vi "X-Parker_Plot.vi"(1 "Route Checking?":bool, 3 "Traverse Name":string, 5 "Coordinate rotation (deg)":dbl format="%.2f", 9 "Points to plot":dbl[][](array[numeric]) format="%.2f", 11 "Work in Tunnel Coordinates?":T1, 13 "Speed Factor":dbl=1.0 min=0.1 max=5.0 format="%.2f") -> (4 "Position Output XYZ":dbl[](array[numeric]) format="%.2f", 15 "Error String":string)   [LabVIEW 2010]
uses:
  Gen Trav/Trav_mode.ctl
  ADAM Serial/Instrument drivers/PARKER X/~subVIs/X-_Channel_Config_Global.vi
  Globals/Trav_pos_global.vi
  ADAM Client/Sub VIs/ADAM Controls/Update_scan_value.ctl
  Gen Trav/Route mapping/Route_mapping_global.vi
  Globals/Preference_global.vi
  Controls/Tunnel_Coordinates.ctl
panel:
  out "Server copy Location":path
  in  "Backlash Compensation?":bool
  out "Log File":path
  out "Achieved Pos In Eng units of all channels":dbl[](array[numeric]) format="%.2f"
  out "Pulses Positon all channels":dbl[](array[numeric])
  out "Counters Reset?":bool
  in  "Mode":T2
  # "X                Y                   Z"
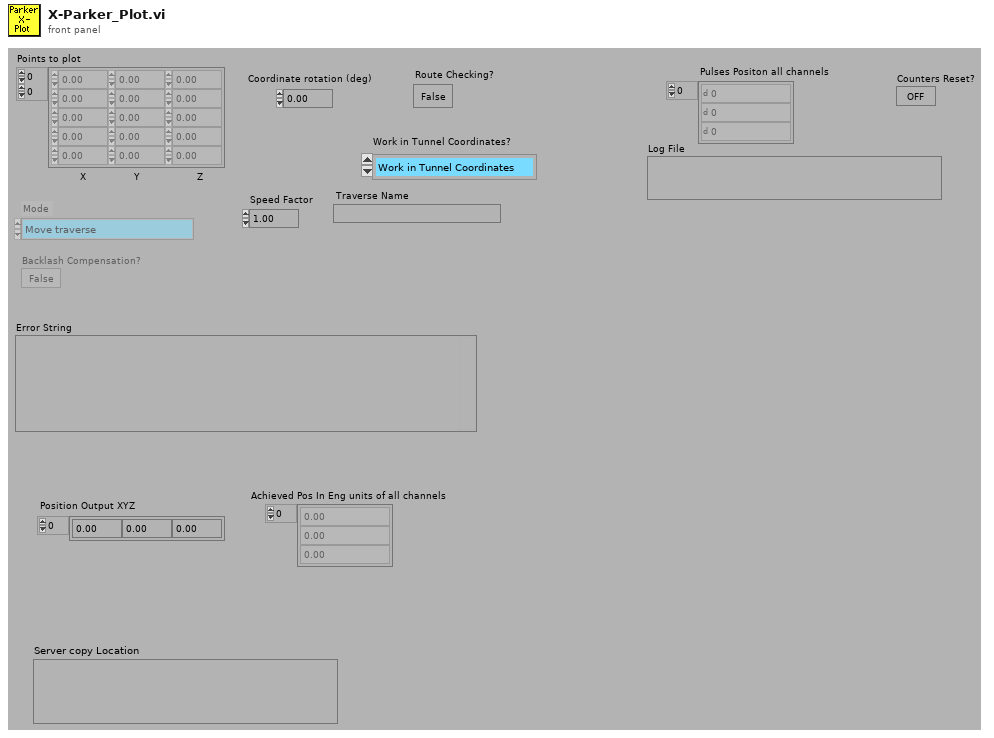
[diagram p1: front panel]
types:
  T1 = typedef "Tunnel_Coordinates.ctl" = enum16{"Work in Tunnel Coordinates", "Work in Model Coordinates"}
  T2 = typedef "Trav_mode.ctl" = enum16{"Move traverse", "Read traverse position", "Teach Position"}
  T3 = enum16{"A-    Acceleration (rps)", "B-    Buffer Status", "C-    Continue", "CG-  Correction Gain", "CR-  Cariage Return", "D-    Distance (pulses)", "DB-  Dead Band (encoder steps)", "DW- Deadband Window (encoder steps)", "E-    Enable Communications", "ER-  Encoder Resolution (steps/rev)", "F-    Disable Communications", "FS-  Encoder Functions Report", "FSA- Incremental/Absolute (0/1)", "FSB- Motor/Encoder Step Mode (0/1)", "FSC- Enable/Disable Position Maint. (1/0)", "FSD- Stop/Continue on Stall (1/0)", "FSE- Activate o/p1 on Stall (1/0)", "FSF- Stop Motion on Trig3 (1/0)", "FSG- Activate o/p2 in Deadband (1/0)", "FSH- Enable Stall Detect (1/0)", "G- Go", "GH- Go Home and Zero (+/-V)", "^H- Delete ", "H- Direction Reverse/CCW/CW (0,1,2)", "IS- Input Status", "K- Kill", "L- Loop (n)", "LD- Limit DISABLE (0-none,1-CW,2-CCW,3-Both)", "LF- Line Feed", "MC- Mode Continuous", "MN- Mode Normal", "MPA- Motor Postion Absolute", "MPI- Motor Position Incremental", "MR- Motor Resolution (Drive Steps/rev)", "N- End of Loop", "O- Output (00,01,10,11)", "OS- Report Homing Setup", "OSA- NO/NC Limits (1/0)", "OSB- Back Up to Home/Edge? (0/1)", "OSC- NO/NC Home Switch (1/0)", "OSD- Enable Encoder Z for Home (0/1)", "OSH- Reference Edge for Home CW/CCW (0/1)", "PR- Report ABSOLUTE Position", "PS- Pause until Continue", "PX- Report Absolute ENCODER Position", "PZ- Zero Absolute Counter", "\"- Quote (17 ASCII +Space)", "Q- Enter/Exit Velocity Profiling (1/0)", "R- Request Indexer Status", "RA- Report Limit Switch Status", "RB- Report Loop, Pause, Shutdown, Trigger Status", "RC- Report Closed Loop Status", "RM- Velocity Streaming Rate Multiplier (000-FFF)", "RV- Report Revision Level", "S- Controlled Stop", "SN- Debounce (1-1000ms)", "SS- Report Software Switch Status", "SSA- Disable RS232 Echo (1/0)", "SSG- Clear/Save Command Buffer on Limit (0/1)", "SSH- Clear/Save Command Buffer on Stop (0/1)", "ST- Shutdown (1/0)", "SV- Servoing Setting (0,1,2,3)", "T- Time Delay (0.01-99999.99)", "TR- Wait for Trigger High/Low/Ignore (1/0/X)", "TS- Report Trigger Status", "U- Pause after Move Until Continue", "V- Velocity (0.01-50.00 revs/sec)", "W1- Report Relative Position <Signed Binary>", "W3- Report Relative Position <Hexadecimal>", "Y- Abort Loop at N", "Z-    Reset to Defaults", "#-    Disable/Set Soft Addresses (0/1-255)"}
  T4 = enum16{"To Traverse Coordinates", "To User Coordinates"}
  T5 = typedef "Update_scan_value.ctl" = cluster{"Channel Name":string, "New Value":dbl}
  T6 = typedef "X-Config_Cluster.ctl" = cluster{"Channel Properties":T7, "Static Drive Configuration":T8}
  T7 = typedef "Ch_Properties.ctl" = cluster{"Channel Name":string, "Vel. Default":dbl, "Acc. Default":dbl, "Vel. Max":dbl, "Vel. Min":dbl, "Acc. Max":dbl, "Acc. Min":dbl, "Pulses/unit":dbl, "Address":u8, "Pulse Offset":i32, "Pos Tolerance":dbl, "Pulses/rev":dbl, "Backlash/Eng units":dbl, "Current Pos":dbl, "Ch Status":enum16{"Active", "Offline", "Simulate"}, "Port Name":string, "Axis Transform mode":string, "Metadata Ch Name":string}
  T8 = typedef "X-_Static_Config.ctl" = cluster{"Correction Gain % (CG)":u16, "Dead Band (DB)":i32, "Dead Band Window (DW)":i32, "Encoder Resolution (ER)":i32, "Step Mode  (FSB)":u16, "Position Maintenance (FSC)":u16, "Stop on Stall (FSD)":u16, "Activate OP1 on stall (FSE)":u16, "Stop on Trigger 3 (FSF)":u16, "OP2 in Deadband (FSG)":u16, "Stall Detect (FSH)":u16, "Limit Disable (LD)":u16, "Motor Resolution (MR)":enum16{"200", "400", "1000", "2000", "4000", "5000", "10000", "12800", "18000", "20000", "21600", "25000", "25400", "25600", "36000", "50000", "278528", "425984", "507904", "614400", "655360", "819200", "1024000"}, "Limit Switch Sense (OSA)":u16, "Home Position (OSB)":u16, "Home Switch Sense (OSC)":u16, "Encoder Z for Home (OSD)":u16, "Reference edge of Home (OSH)":u16, "RS232 Echo Control (SSA)":u16, "Buffer at Limit (SSG)":u16, "Buffer at Stop (SSH)":u16, "Indexer Mode  (FSA)":u16}
  T9 = typedef "Box_size.ctl" = cluster{"Max":dbl, "Min":dbl}[]
  T10 = typedef "Exclude_cluster.ctl" = cluster{"Sizes":T9, "Name":string, "Exclude Type":T11}
  T11 = typedef "Exclusion_type.ctl" = enum16{"Exclude completely", "Allow only vertical moves"}
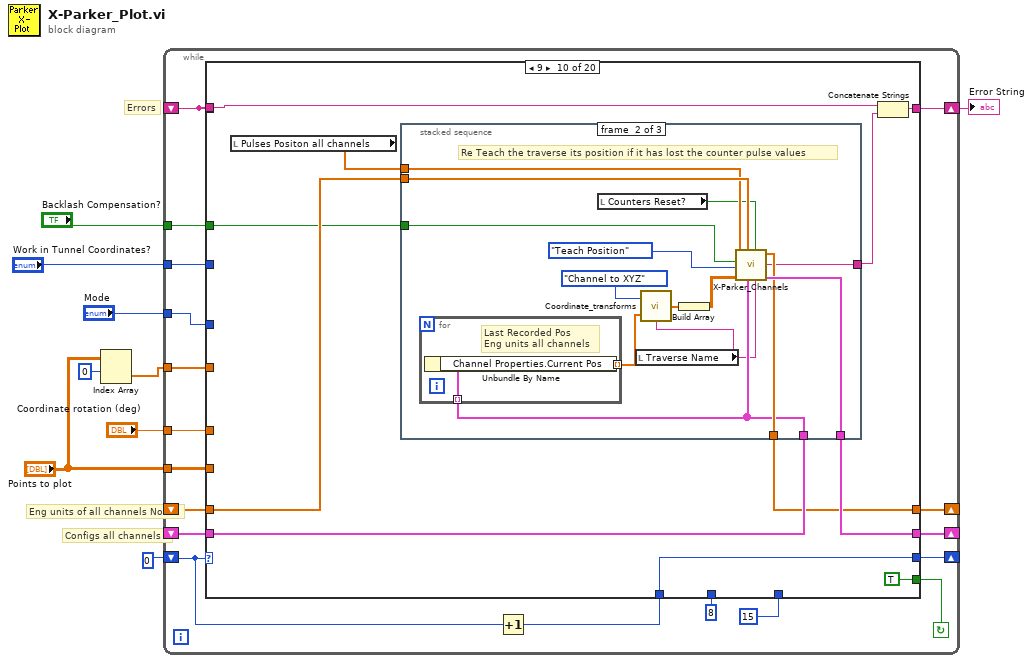
[diagram p0: block diagram]
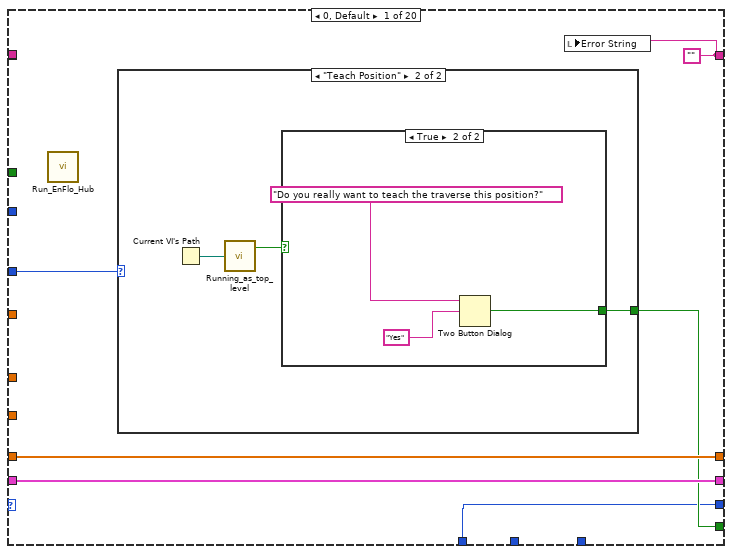
[diagram p2: hidden frame]
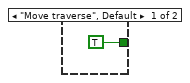
[diagram p3: hidden frame]
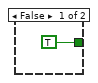
[diagram p4: hidden frame]
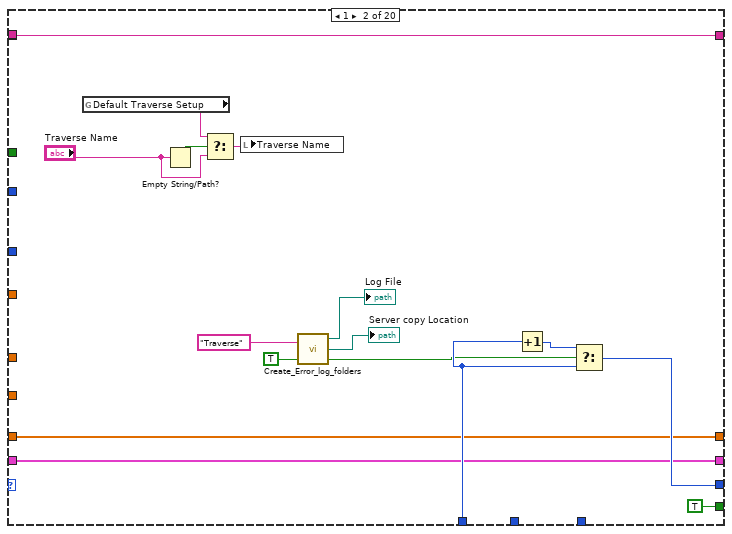
[diagram p5: hidden frame]
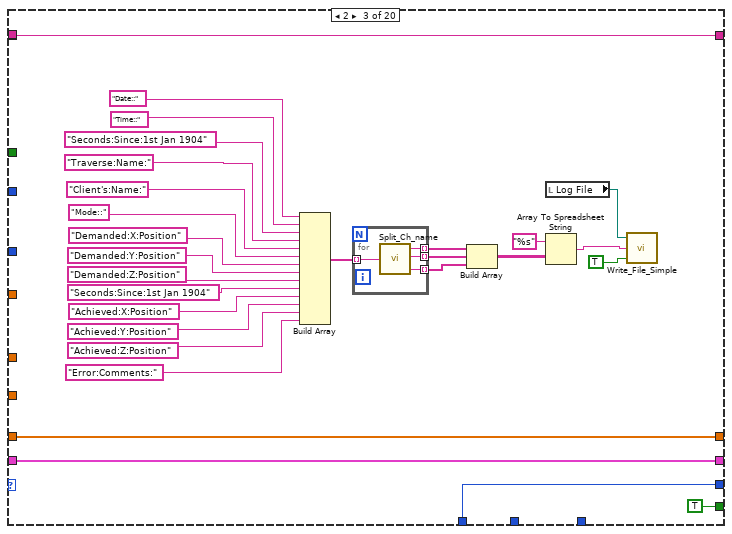
[diagram p6: hidden frame]
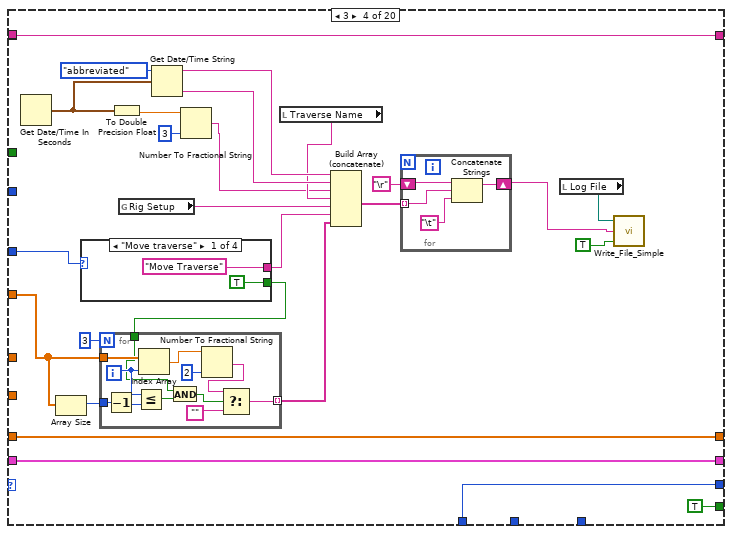
[diagram p7: hidden frame]
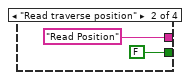
[diagram p8: hidden frame]
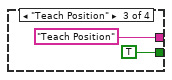
[diagram p9: hidden frame]
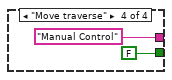
[diagram p10: hidden frame]
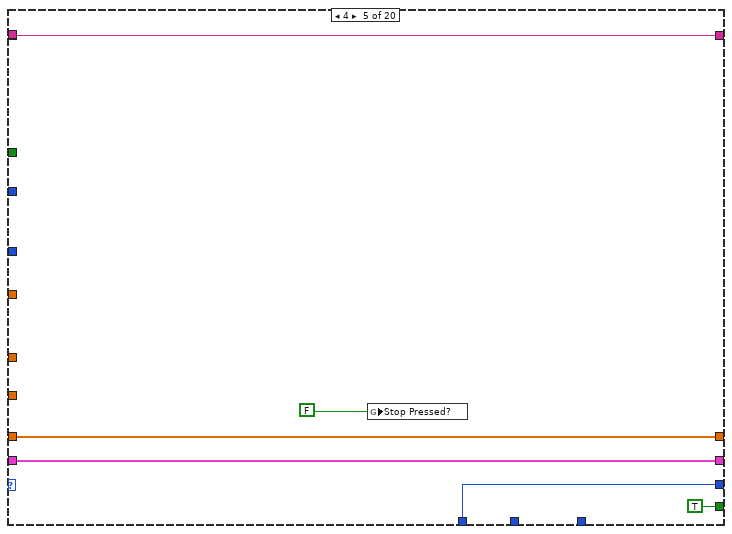
[diagram p11: hidden frame]
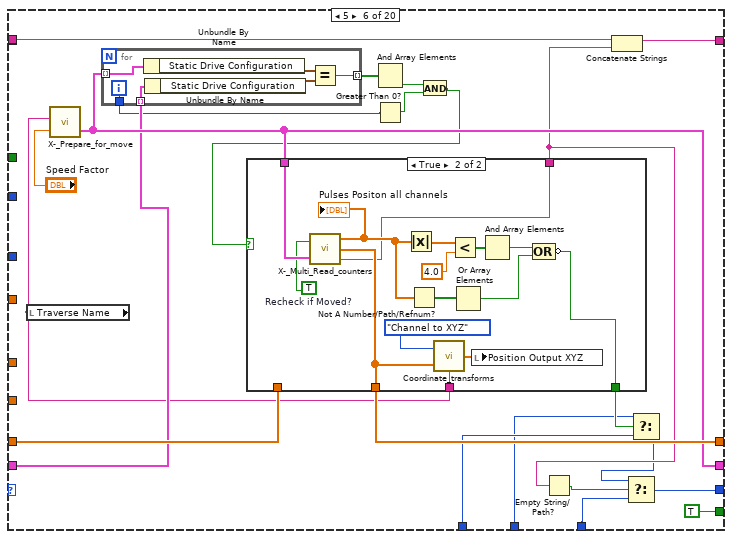
[diagram p12: hidden frame]
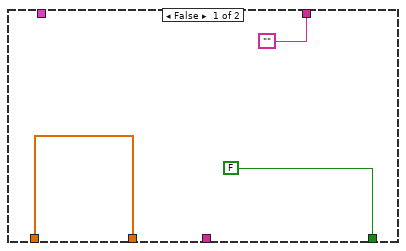
[diagram p13: hidden frame]
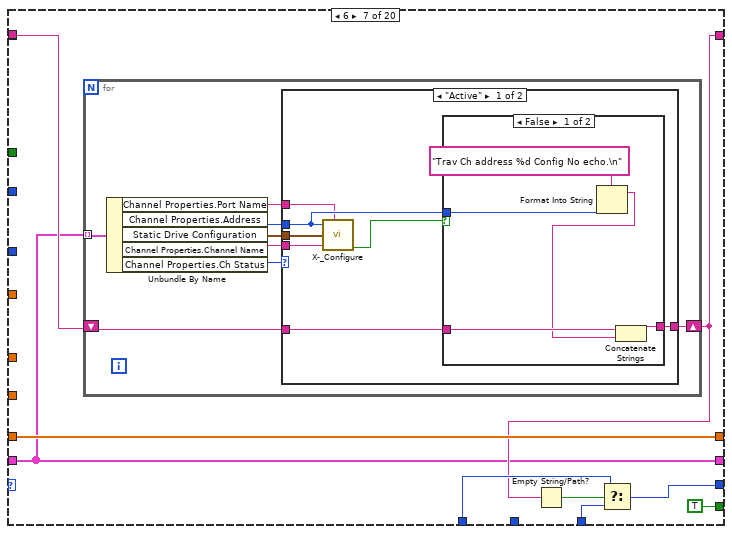
[diagram p14: hidden frame]
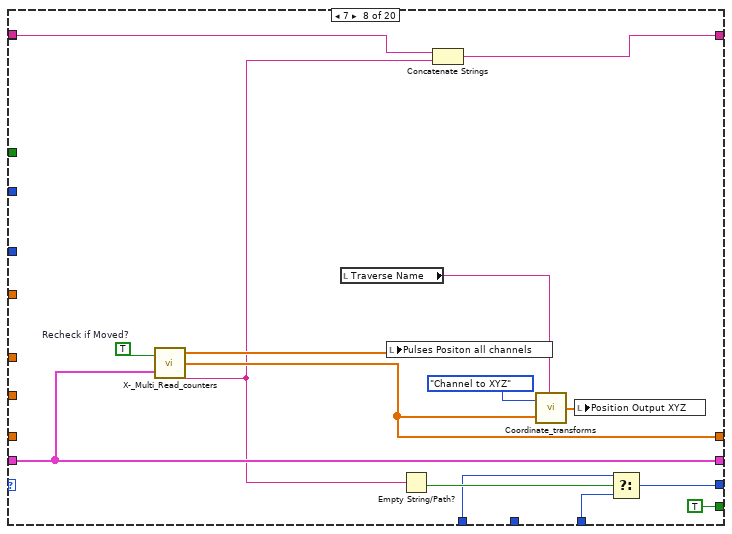
[diagram p17: hidden frame]
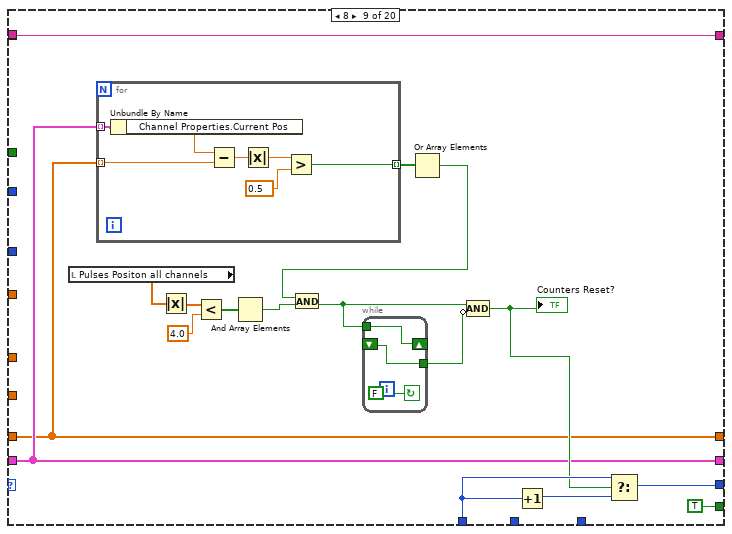
[diagram p18: hidden frame]
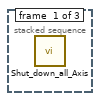
[diagram p19: hidden frame]
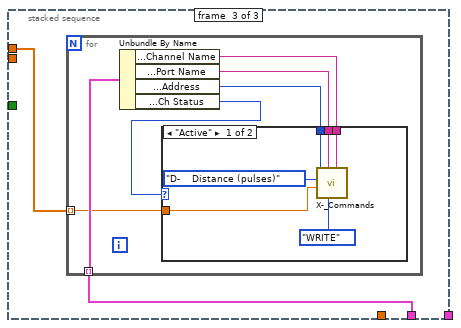
[diagram p20: hidden frame]
diagram:
  # "Errors"
  # "Eng units of all channels Now"
  # "Configs all channels"
  n1 = Index Array(array="Points to plot", index (row)=0) -> (element=w2:dbl[])  [unwired: 1 in]
  n2 = while {
    tunnel: "Backlash Compensation?" -> [w13]
    tunnel: w2 -> [w17]
    shift-left: _ -> [w14]
    shift-right: [w18] -> w7
    shift-left: _ -> [w19]
    shift-right: [w20] -> _
    shift-left: _ -> [w21]
    shift-right: [w22] -> _
    shift-left: 0 -> [w25]
    shift-right: [w23] -> _
    tunnel: "Mode" -> [w27]
    tunnel: "Coordinate rotation (deg)" -> [w12]
    tunnel: "Work in Tunnel Coordinates?" -> [w11]
    tunnel: "Points to plot" -> [w10]
    stop <- w26 continue-if-true
    n3 = Increment(x=w25) -> (x+1=w24:i32)
    n4 = case shown="9" w25 {
      tunnel: w27 -> [w33 _ _ w108 _ _ _ _ _ _ w311 _ w389 w405 _ _ _ w477 _ w533]
      tunnel: [w30 TRUE ("T button?") TRUE ("T button?") TRUE ("T button?") TRUE TRUE ("T button?") TRUE ("T button?") TRUE ("T button?") TRUE TRUE TRUE ("T button?") TRUE ("T button?") TRUE TRUE TRUE ("T button?") TRUE ("T button?") TRUE ("T button?") w479 TRUE FALSE] -> w26
      tunnel: w24 -> [w29 w56 w65 w113 w140 w164 w197 w225 w250 w266 w310 w343 w380 w407 w429 w443 w472 w476 w511 w540]
      tunnel: [w29 w54 w65 w113 w140 w147 w196 w223 w248 w266 w309 w344 w380 w406 w429 w441 w472 w475 w511 w540] -> w23
      tunnel: [w31 w51 w67 w115 w142 w162 w192 w237 w244 w275 w307 w346 w374 w404 w431 w455 w474 w482 w509 w538] -> w22
      tunnel: w21 -> [w31 w51 w67 w115 w142 w161 w192 w237 w244 w274 w307 w346 w387 w404 w431 w455 w474 w482 w509 w538]
      tunnel: [w32 w52 w66 w114 w143 w167 w200 w232 w243 w271 w306 w333 w381 w410 w430 w454 w473 w483 w512 w541] -> w20
      tunnel: w19 -> [w32 w52 w66 w114 w143 w166 w200 _ w243 w272 w306 w333 w376 w410 w430 w454 w473 w483 w512 w541]
      tunnel: [w28 w50 w63 w105 w144 w152 w193 w228 w247 w268 w312 w337 w383 w408 w427 w445 w470 w478 w505 w534] -> w18
      tunnel: w14 -> [_ w50 w63 w105 w144 w153 w194 w229 w247 w270 w312 _ w384 w408 w427 w445 w470 w481 w507 w536]
      tunnel: w17 -> [_ _ _ w102 _ _ _ _ _ _ _ _ _ _ _ _ _ _ w503 _]
      tunnel: 15 ("f") -> [_ _ _ _ _ w148 w195 w224 _ _ _ w339 _ _ _ _ _ _ _ _]
      tunnel: 8 ("t") -> [_ _ _ _ _ w163 _ _ _ _ _ _ _ _ _ _ _ _ _ _]
      tunnel: w14 -> [_ _ _ _ _ _ _ _ _ _ _ w340 _ _ _ _ _ _ _ _]
      tunnel: w13 -> [_ _ _ _ _ _ _ _ _ w265 _ _ w375 w399 _ _ _ _ _ _]
      tunnel: w12 -> [_ _ _ _ _ _ _ _ _ _ _ w332 w372 _ _ _ _ _ w504 w531]
      tunnel: w11 -> [_ _ _ _ _ _ _ _ _ _ _ _ w373 _ _ _ _ _ w501 w529]
      tunnel: w10 -> [_ _ _ _ _ _ _ _ _ _ _ w325 w371 _ _ _ _ _ _ _]
      frame 0, Default {
        w28 = ""
        n5 = call "Run_EnFlo_Hub.vi"() -> ()  [unwired: 8 in]
        n6 = case shown="\"Teach Position\"" w33 {
          tunnel: [TRUE ("T button?") w35] -> w30
          frame "Move traverse", Default {
          }
          frame "Teach Position" {
            n7 = Current VI's Path() -> (path=w37:path)
            n8 = call "Running_as_top_level.vi"("Vi path name"=w37) -> ("Top Level"=w36:bool)  [unwired: 1 out]
            n9 = case shown="True" w36 {
              tunnel: [TRUE ("T button?") w39] -> w35
              frame False {
              }
              frame True {
                n10 = Two Button Dialog(message="Do you really want to teach the traverse this position?", 2:"Yes" ("T button name (\"OK\")")) -> (T button?=w39:bool)  [unwired: 1 in]
              }
            }
          }
        }
        n11 = local write "Error String"(w28) -> ()
      }
      frame 1 {
        n12 = global read "Trav_pos_global.vi" "Default Traverse Setup"() -> (w47:string)
        n13 = Empty String/Path?(string/path="Traverse Name") -> (empty?=w45:bool)
        n14 = Select(t=w47, s=w45, f="Traverse Name") -> (s? t:f=w44:string)
        n15 = local write "Traverse Name"(w44) -> ()
        n16 = call "Create_Error_log_folders.vi"("Per Day Log File?"=TRUE, "Log Filename"="Traverse" ("Input Element")) -> ("exists?"=w48:bool, "Server copy Location"=→"Server copy Location":path, "Local Log File"=→"Log File":path)  [unwired: 1 in]
        n17 = Increment(x=w56) -> (x+1=w55:i32)
        n18 = Select(t=w55, s=w48, f=w56) -> (s? t:f=w54:i32)
      }
      frame 2 {
        n19 = Build Array("Date::", "Time::", "Seconds:Since:1st Jan 1904", "Traverse:Name:", "Client's:Name:", "Mode::", "Demanded:X:Position", "Demanded:Y:Position", "Demanded:Z:Position", "Seconds:Since:1st Jan 1904", "Achieved:X:Position", "Achieved:Y:Position", "Achieved:Z:Position", "Error:Comments:") -> (w70:string[])
        n20 = for {
          tunnel: w70 -> [w89] mode=indexing
          tunnel: [w88] -> w71 mode=indexing
          tunnel: [w87] -> w72 mode=indexing
          tunnel: [w86] -> w73 mode=indexing
          n21 = call "Split_Ch_name.vi"("Ch name"=w89) -> ("Top level"=w88:string, "Middle"=w87:string, "Low level"=w86:string)
        }
        n22 = Build Array(w71, w72, w73) -> (w68:string[][])
        n23 = local read "Log File"() -> (w59:path)
        n24 = Array To Spreadsheet String(array=w68, 3:"%s" ("format string")) -> (spreadsheet string=w60:string)  [unwired: 1 in]
        n25 = call "Write_File_Simple.vi"("append to file? (new file:F)"=TRUE, "character string"=w60, "file path"=w59) -> ()  [unwired: 2 out]
      }
      frame 3 {
        n26 = Get Date/Time In Seconds() -> (seconds since 1Jan1904=w94:timestamp)
        n27 = Array Size(array=w102) -> (size(s)=w103:i32)
        n28 = case shown="\"Move traverse\"" w108 {
          tunnel: ["Move Traverse" "Read Position" "Teach Position" "Manual Control"] -> w109
          tunnel: [TRUE FALSE TRUE FALSE] -> w99
          frame "Move traverse" {
          }
          frame "Read traverse position" {
          }
          frame "Teach Position" {
          }
          frame "Move traverse" {
          }
        }
        n29 = for {
          N: 3 -> [_]
          tunnel: w102 -> [w127]
          tunnel: w103 -> [w124]
          tunnel: [w120] -> w100 mode=indexing
          tunnel: w99 -> [w116]
          i -> [w122]
          n30 = Decrement(x=w124) -> (x-1=w123:i32)
          n31 = Less Or Equal?(x=w122, y=w123) -> (x <= y?=w118:bool)
          n32 = Index Array(array=w127, index=w122) -> (element=w126:dbl)
          n33 = And(x=w116, y=w118) -> (x .and. y?=w117:bool)
          n34 = Number To Fractional String(number=w126, precision (6)=i16 2) -> (F-format string=w121:string)  [unwired: 2 in]
          n35 = Select(t=w121, s=w117, f="") -> (s? t:f=w120:string)
        }
        n36 = To Double Precision Float(number=w94) -> (double precision float=w93:dbl)
        n37 = global read "Preference_global.vi" "Rig Setup"() -> (w90:string)
        n38 = Get Date/Time String(date format (0)=enum16{"short", "long", "abbreviated"}."abbreviated", seconds (now)=w94) -> (date string=w111:string, time string=w110:string)  [unwired: 1 in]
        n39 = Number To Fractional String(number=w93, precision (6)=i16 3) -> (F-format string=w91:string)  [unwired: 2 in]
        n40 = local read "Traverse Name"() -> (w95:string)
        n41 = Build Array (concatenate)(w111, w110, w91, w95, w90, w109, w100) -> (w106:string[])
        n42 = for {
          shift-right: [w130] -> w96
          shift-left: "\r" -> [w131]
          tunnel: w106 -> [w129] mode=indexing
          n43 = Concatenate Strings(w131, w129, "\t") -> (w130:string)
        }
        n44 = local read "Log File"() -> (w97:path)
        n45 = call "Write_File_Simple.vi"("append to file? (new file:F)"=TRUE, "character string"=w96, "file path"=w97) -> ()  [unwired: 2 out]
      }
      frame 4 {
        n46 = global write "X-_Channel_Config_Global.vi" "Stop Pressed?"(FALSE) -> ()
      }
      frame 5 {
        n47 = local read "Traverse Name"() -> (w155:string)
        n48 = call "X-_Prepare_for_move.vi"("Speed Factor"="Speed Factor", "Traverse Name"=w155) -> ("Matched Configurations"=w162:T6[])  [unwired: 1 in]
        n49 = for {
          tunnel: w162 -> [w173] mode=indexing
          tunnel: w161 -> [w172] mode=indexing
          tunnel: [w169] -> w160 mode=indexing
          tunnel: [w168] -> w159
          i -> [w168]
          n50 = Unbundle By Name(w173) -> ("Static Drive Configuration"=w171:T8)
          n51 = Unbundle By Name(w172) -> ("Static Drive Configuration"=w170:T8)
          n52 = Equal?(x=w171, y=w170) -> (x = y?=w169:bool)
        }
        n53 = And Array Elements(Boolean array=w160) -> (logical AND=w157:bool)
        n54 = Greater Than 0?(x=w159) -> (x > 0?=w158:bool)
        n55 = And(x=w157, y=w158) -> (x .and. y?=w156:bool)
        n56 = case shown="True" w156 {
          tunnel: w162 -> [_ w191]
          tunnel: [w176 w181] -> w167
          tunnel: w166 -> [w176 _]
          tunnel: [FALSE w183] -> w165
          tunnel: w155 -> [_ w179]
          tunnel: ["" w177] -> w151
          frame False {
          }
          frame True {
            w178 = TRUE  # Recheck if Moved?
            n57 = call "X-_Multi_Read_counters.vi"("Recheck if Moved?"=w178, "Matched Configurations"=w191) -> ("Pulses"=w186:dbl[], "Eng units"=w181:dbl[], "Error String"=w177:string)
            "Pulses Positon all channels" <- w186
            n58 = Absolute Value(x=w186) -> (abs(x)=w190:dbl[])
            n59 = Not A Number/Path/Refnum?(number/path/refnum=w186) -> (NaN/Path/Refnum?=w185:bool[])
            n60 = call "Coordinate_transforms.vi"("Traverse Name"=w179, "Input"=w181, "Mode"=enum16{"XYZ to Channel", "Channel to XYZ"}."Channel to XYZ") -> ("Output"=w180:dbl[])
            n61 = Less?(x=w190, y=4.0 ("Achieved Position")) -> (x < y?=w188:bool[])
            n62 = Or Array Elements(Boolean array=w185) -> (logical OR=w184:bool)
            n63 = local write "Position Output XYZ"(w180) -> ()
            n64 = And Array Elements(Boolean array=w188) -> (logical AND=w187:bool)
            n65 = Compound Arithmetic op=OR(w187, w184) -> (invert w183:bool)
          }
        }
        n66 = Empty String/Path?(string/path=w151) -> (empty?=w150:bool)
        n67 = Concatenate Strings(w153, w151) -> (w152:string)
        n68 = Select(t=w163, s=w165, f=w164) -> (s? t:f=w149:i32)
        n69 = Select(t=w149, s=w150, f=w148) -> (s? t:f=w147:i32)
      }
      frame 6 {
        n70 = for {
          tunnel: w192 -> [w208] mode=indexing
          shift-right: [w201] -> w193
          shift-left: w194 -> [w202]
          n71 = Unbundle By Name(w208) -> ("Channel Properties.Port Name"=w203:string, "Channel Properties.Address"=w207:u8, "Static Drive Configuration"=w206:T8, "Channel Properties.Channel Name"=w205:string, "Channel Properties.Ch Status"=w204:enum16{"Active", "Offline", "Simulate"})
          n72 = case shown="\"Active\"" w204 {
            tunnel: w207 -> [w213 _]
            tunnel: w206 -> [w215 _]
            tunnel: w205 -> [w214 _]
            tunnel: w203 -> [w212 _]
            tunnel: w202 -> [w210 w222]
            tunnel: [w209 w222] -> w201
            frame "Active" {
              n73 = call "X-_Configure.vi"("Address"=w213, "Port Name"=w212, "Static Drive Configuration"=w215, "Channel Name"=w214) -> ("Good Echo"=w211:bool)  [unwired: 4 in]
              n74 = case shown="False" w211 {
                tunnel: w213 -> [w220 _]
                tunnel: w210 -> [w218 w221]
                tunnel: [w217 w221] -> w209
                frame False {
                  n75 = Format Into String(format string="Trav Ch address %d Config No echo.\n" ("Format String"), w220) -> (resulting string=w216:string)  [unwired: 2 in, 1 out]
                  n76 = Concatenate Strings(w218, w216) -> (w217:string)
                }
                frame True {
                }
              }
            }
            frame "Offline", Default {
            }
          }
        }
        n77 = Empty String/Path?(string/path=w193) -> (empty?=w198:bool)
        n78 = Select(t=w197, s=w198, f=w195) -> (s? t:f=w196:i32)
      }
      frame 7 {
        w230 = TRUE  # Recheck if Moved?
        n79 = call "X-_Multi_Read_counters.vi"("Recheck if Moved?"=w230, "Matched Configurations"=w237) -> ("Pulses"=w235:dbl[], "Eng units"=w232:dbl[], "Error String"=w226:string)
        n80 = local read "Traverse Name"() -> (w231:string)
        n81 = local write "Pulses Positon all channels"(w235) -> ()
        n82 = Empty String/Path?(string/path=w226) -> (empty?=w227:bool)
        n83 = Concatenate Strings(w229, w226) -> (w228:string)
        n84 = call "Coordinate_transforms.vi"("Traverse Name"=w231, "Input"=w232, "Mode"=enum16{"XYZ to Channel", "Channel to XYZ"}."Channel to XYZ") -> ("Output"=w233:dbl[])
        n85 = local write "Position Output XYZ"(w233) -> ()
        n86 = Select(t=w225, s=w227, f=w224) -> (s? t:f=w223:i32)
      }
      frame 8 {
        n87 = local read "Pulses Positon all channels"() -> (w238:dbl[])
        n88 = for {
          tunnel: w244 -> [w264] mode=indexing
          tunnel: w243 -> [w262] mode=indexing
          tunnel: [w258] -> w241 mode=indexing
          n89 = Unbundle By Name(w264) -> ("Channel Properties.Current Pos"=w263:dbl)
          n90 = Subtract(x=w263, y=w262) -> (x-y=w261:dbl)
          n91 = Absolute Value(x=w261) -> (abs(x)=w260:dbl)
          n92 = Greater?(x=w260, y=0.5) -> (0:w258:bool)
        }
        n93 = Absolute Value(x=w238) -> (abs(x)=w254:dbl[])
        n94 = Less?(x=w254, y=4.0 ("Achieved Position")) -> (x < y?=w252:bool[])
        n95 = And Array Elements(Boolean array=w252) -> (logical AND=w242:bool)
        n96 = Or Array Elements(Boolean array=w241) -> (logical OR=w240:bool)
        n97 = And(x=w240, y=w242) -> (x .and. y?=w239:bool)
        n98 = while {
          tunnel: [w256] -> w246
          tunnel: w239 -> [w257]
          shift-left: _ -> [w256]
          shift-right: [w257] -> _
          stop <- FALSE continue-if-true
        }
        n99 = Compound Arithmetic op=AND(w239, invert w246) -> (w245:bool)
        "Counters Reset?" <- w245
        n100 = Increment(x=w250) -> (x+1=w249:i32)
        n101 = Select(t=w250, s=w245, f=w249) -> (s? t:f=w248:i32)
      }
      frame 9 {
        n102 = local read "Pulses Positon all channels"() -> (w273:dbl[])
        n103 = stacked-sequence {
          tunnel: w273 -> [_ w281 w292]
          tunnel: [_ w289 _] -> w275
          tunnel: w272 -> [_ w288 _]
          tunnel: [_ w287 _] -> w271
          tunnel: w274 -> [_ w283 w293]
          tunnel: [_ w286 _] -> w269
          tunnel: w265 -> [_ w277 _]
          frame #0 {
            n104 = call "Shut_down_all_Axis.vi"() -> ()  [unwired: 1 in]
          }
          frame #1 {
            # "Re Teach the traverse its position if it has lost the counter pulse values"
            n105 = for {
              tunnel: [w291] -> w282 mode=indexing
              tunnel: w283 -> [w290] mode=indexing
              # "Last Recorded Pos\nEng units all channels"
              n106 = Unbundle By Name(w290) -> ("Channel Properties.Current Pos"=w291:dbl)
            }
            n107 = local read "Counters Reset?"() -> (w279:bool)
            n108 = local read "Traverse Name"() -> (w278:string)
            n109 = call "Coordinate_transforms.vi"("Traverse Name"=w278, "Input"=w282, "Mode"=enum16{"XYZ to Channel", "Channel to XYZ"}."Channel to XYZ") -> ("Output"=w284:dbl[])
            n110 = Build Array(w284) -> (w276:dbl[][])
            n111 = call "X-Parker_Channels.vi"("Traverse Name"=w278, "Counters Reset?"=w279, "Matched Configurations all Channels In"=w283, "Current Pos In Eng units of all channels"=w288, "Position Steps"=w276, "Mode"=Trav_mode."Teach Position", "Backlash Compensation?"=w277, "Current Pulses positions for all channels"=w281) -> ("Matched Configurations Out"=w289:T6[], "Error String"=w286:string, "Achieved Pos In Eng units of all channels"=w287:dbl[])  [unwired: 1 in]
          }
          frame #2 {
            n112 = for {
              tunnel: w293 -> [w299] mode=indexing
              tunnel: w292 -> [w296] mode=indexing
              n113 = Unbundle By Name(w299) -> ("Channel Properties.Channel Name"=w294:string, "Channel Properties.Port Name"=w295:string, "Channel Properties.Address"=w298:u8, "Channel Properties.Ch Status"=w297:enum16{"Active", "Offline", "Simulate"})
              n114 = case shown="\"Active\"" w297 {
                tunnel: w295 -> [w305 _]
                tunnel: w294 -> [w304 _]
                tunnel: w298 -> [w301 _]
                tunnel: w296 -> [w300 _]
                frame "Active" {
                  n115 = call "X-_Commands.vi"("Channel Name"=w304, "R/W"=enum16{"READ", "WRITE"}."WRITE", "Port Name"=w305, "Numeric Value"=w300, "COMMAND"=T3."D-    Distance (pulses)", "Address"=w301) -> ()  [unwired: 3 in, 2 out]
                }
                frame "Offline", Default {
                }
              }
            }
          }
        }
        n116 = Concatenate Strings(w270, w269) -> (w268:string)
      }
      frame 10 {
        n117 = case shown="\"Move traverse\"" w311 {
          tunnel: w310 -> [w313 w320]
          tunnel: [w315 w319] -> w309
          frame "Move traverse" {
            n118 = Increment(x=w313) -> (x+1=w314:i32)
            n119 = case shown="True" "Route Checking?" {
              tunnel: [w317 w318] -> w315
              tunnel: w314 -> [w317 _]
              tunnel: w313 -> [_ w318]
              frame False {
              }
              frame True {
              }
            }
          }
          frame "Read traverse position", Default {
            n120 = Increment(x=w320) -> (x+1=w319:i32)
          }
        }
      }
      frame 11 {
        w328 = 0.1  # Reduce by
        n121 = global read "Route_mapping_global.vi" "Probe Volume"() -> (w327:T9)
        n122 = local read "Traverse Name"() -> (w334:string)
        n123 = for {
          tunnel: w327 -> [w369] mode=indexing
          tunnel: [w368] -> w326 mode=indexing
          tunnel: w328 -> [w363]
          n124 = Unbundle By Name(w369) -> ("Max"=w367:dbl, "Min"=w365:dbl)
          n125 = Subtract(x=w367, y=w363) -> (x-y=w366:dbl)
          n126 = Add(x=w363, y=w365) -> (x+y=w364:dbl)
          n127 = Bundle By Name(cluster=w369, "Max"=w366, "Min"=w364) -> (w368:cluster{"Max":dbl, "Min":dbl})
        }
        n128 = global read "Route_mapping_global.vi" "Entire Space"() -> (w329:T9)
        n129 = global read "Route_mapping_global.vi" "Exclude Array"() -> (w330:T10[])
        n130 = call "Coordinate_transforms.vi"("Traverse Name"=w334, "Input"=w333, "Mode"=enum16{"XYZ to Channel", "Channel to XYZ"}."Channel to XYZ") -> ("Output"=w335:dbl[])
        n131 = Array Size(array=w325) -> (size(s)=w324:i32[])
        n132 = Index Array(array=w324, index=0) -> (element=w322:i32)
        n133 = call "Coordinate_rotation.vi"("Input Position"=w335, "Coordinate rotation (deg)"=w332, "Mode"=T4."To User Coordinates") -> ("Output Position"=w341:dbl[])
        n134 = Decrement(x=w322) -> (x-1=w321:i32)
        n135 = while {
          tunnel: w341 -> [w361]
          tunnel: w325 -> [w359] mode=indexing
          tunnel: w334 -> [w358]
          tunnel: w332 -> [w356]
          tunnel: [w352] -> w331
          tunnel: w330 -> [w355]
          tunnel: w329 -> [w354]
          tunnel: w326 -> [w353]
          tunnel: w321 -> [w350]
          i -> [w351]
          stop <- w347 continue-if-true
          w357 = FALSE  # Full Check
          n136 = Less?(x=w351, y=w350) -> (x < y?=w348:bool)
          n137 = call "Coordinate_rotation.vi"("Input Position"=w359, "Coordinate rotation (deg)"=w356, "Mode"=T4."To User Coordinates") -> ("Output Position"=w360:dbl[])
          n138 = call "Check_Traverse_move.vi"("Current position"=w361, "Traverse Name"=w358, "Full Check"=w357, "New Position"=w360, "Coordinate rotation (deg)"=w356, "Probe Volume"=w353, "Entire Space"=w354, "Exclude Array"=w355) -> ("Error Comments"=w352:string)  [unwired: 5 in, 2 out]
          n139 = Empty String/Path?(string/path=w352) -> (empty?=w349:bool)
          n140 = And(x=w349, y=w348) -> (x .and. y?=w347:bool)
        }
        n141 = Empty String/Path?(string/path=w331) -> (empty?=w338:bool)
        n142 = Select(t=w343, s=w338, f=w339) -> (s? t:f=w344:i32)
        n143 = Concatenate Strings(w340, w331) -> (w337:string)
      }
      frame 12 {
        w378 = FALSE  # Counters Reset?
        n144 = case shown="\"Work in Model Coordinates\"" w373 {
          tunnel: w372 -> [_ w393]
          tunnel: w371 -> [w390 w392]
          tunnel: [w390 w391] -> w370
          frame "Work in Tunnel Coordinates" {
          }
          frame "Work in Model Coordinates" {
            n145 = for {
              tunnel: w392 -> [w396] mode=indexing
              tunnel: [w395] -> w391 mode=indexing
              tunnel: w393 -> [w394]
              n146 = call "Coordinate_rotation.vi"("Input Position"=w396, "Coordinate rotation (deg)"=w394, "Mode"=T4."To Traverse Coordinates") -> ("Output Position"=w395:dbl[])
            }
          }
        }
        n147 = local read "Pulses Positon all channels"() -> (w388:dbl[])
        n148 = local read "Traverse Name"() -> (w377:string)
        n149 = call "X-Parker_Channels.vi"("Traverse Name"=w377, "Counters Reset?"=w378, "Matched Configurations all Channels In"=w387, "Current Pos In Eng units of all channels"=w376, "Position Steps"=w370, "Mode"=w389, "Backlash Compensation?"=w375, "Current Pulses positions for all channels"=w388) -> ("Matched Configurations Out"=w374:T6[], "Error String"=w382:string, "Achieved Pos In Eng units of all channels"=w381:dbl[])  [unwired: 1 in]
        "Achieved Pos In Eng units of all channels" <- w381
        n150 = call "Coordinate_transforms.vi"("Traverse Name"=w377, "Input"=w381, "Mode"=enum16{"XYZ to Channel", "Channel to XYZ"}."Channel to XYZ") -> ("Output"=→"Position Output XYZ":dbl[])
        n151 = Concatenate Strings(w384, w382) -> (w383:string)
      }
      frame 13 {
        n152 = local read "Position Output XYZ"() -> (w402:dbl[])
        n153 = case shown="\"Read traverse position\"" w405 {
          tunnel: w402 -> [_ _ _ _]
          frame "Move traverse" {
          }
          frame "Read traverse position" {
          }
          frame "Move traverse" {
          }
          frame "Teach Position" {
            n154 = local write "Mode"(Trav_mode."Read traverse position" ("Mode")) -> ()
          }
        }
        n155 = for {
          tunnel: w404 -> [w418] mode=indexing
          tunnel: T5 {"Channel Name"="", "New Value"=0.0} ("Update Scan Value Cluster") -> [w416]
          tunnel: w402 -> [w414] mode=indexing
          shift-right: [w412] -> w400
          shift-left: T5[] [] -> [w413]
          n156 = Unbundle By Name(w418) -> ("Channel Properties.Metadata Ch Name"=w415:string)
          n157 = Empty String/Path?(string/path=w415) -> (empty?=w417:bool)
          n158 = case shown="False" w417 {
            tunnel: w416 -> [w424 _]
            tunnel: w415 -> [w423 _]
            tunnel: w414 -> [w422 _]
            tunnel: w413 -> [w420 w425]
            tunnel: [w419 w425] -> w412
            frame False {
              n159 = Bundle By Name(cluster=w424, "Channel Name"=w423, "New Value"=w422) -> (w421:T5)
              n160 = Build Array (concatenate)(w420, w421) -> (w419:T5[])
            }
            frame True {
            }
          }
        }
        n161 = global write "X-_Channel_Config_Global.vi" "Run Emergency stop loop"(FALSE ("Run Emergency stop loop")) -> ()
        n162 = Increment(x=w407) -> (x+1=w406:i32)
        n163 = Not(x=w399) -> (.not. x?=w398:bool)
        n164 = call "Update_Current_Value_client.vi"("Don't Bother with check?"=w398, "Update array in"=w400) -> ()
      }
      frame 14 {
      }
      frame 15 {
        n165 = local read "Position Output XYZ"() -> (w449:dbl[])
        n166 = Array Size(array=w449) -> (size(s)=w448:i32)
        n167 = Get Date/Time In Seconds() -> (seconds since 1Jan1904=w440:timestamp)
        n168 = for {
          N: 3 -> [_]
          tunnel: w449 -> [w469]
          tunnel: w448 -> [w466]
          tunnel: [w461] -> w447 mode=indexing
          i -> [w464]
          n169 = Decrement(x=w466) -> (x-1=w465:i32)
          n170 = Less Or Equal?(x=w464, y=w465) -> (x <= y?=w463:bool)
          n171 = Index Array(array=w469, index=w464) -> (element=w468:dbl)
          n172 = Number To Fractional String(number=w468, precision (6)=i16 2) -> (F-format string=w462:string)  [unwired: 2 in]
          n173 = Select(t=w462, s=w463, f="") -> (s? t:f=w461:string)
        }
        n174 = To Double Precision Float(number=w440) -> (double precision float=w433:dbl)
        n175 = Number To Fractional String(number=w433, precision (6)=i16 3) -> (F-format string=w432:string)  [unwired: 2 in]
        n176 = call "Remove_unprintable_Char.vi"("Input String"=w445) -> ("Output String"=w446:string)
        n177 = Build Array (concatenate)(w432, w447, w446) -> (w451:string[])
        n178 = local read "Route Checking?"() -> (w444:bool)
        n179 = for {
          shift-right: [w458] -> w437
          shift-left: "" -> [w459]
          tunnel: w451 -> [w457] mode=indexing
          n180 = Concatenate Strings(w459, w457, "\t") -> (w458:string)
        }
        n181 = Increment(x=w443) -> (x+1=w442:i32)
        n182 = local read "Server copy Location"() -> (w435:path)
        n183 = local read "Log File"() -> (w438:path)
        n184 = Select(t=w442, s=w444, f=w443) -> (s? t:f=w441:i32)
        n185 = call "Write_File_Simple.vi"("append to file? (new file:F)"=TRUE, "character string"=w437, "file path"=w438) -> ("file path Out"=w436:path)  [unwired: 1 out]
        n186 = call "Updated_File_Copy.vi"("Target Path"=w435, "Source Path"=w436) -> ()  [unwired: 1 in, 1 out]
      }
      frame 16 {
      }
      frame 17 {
        n187 = local read "Position Output XYZ"() -> (w484:dbl[])
        n188 = local read "Counters Reset?"() -> (w485:bool)
        n189 = Index Array(array=w484, index=2) -> (element=w490:dbl)
        n190 = Index Array(array=w484, index=0) -> (element=w492:dbl)
        n191 = Index Array(array=w484, index=1) -> (element=w491:dbl)
        n192 = Format Into String(format string="X= %.2f\tY= %.2f\tZ= %.2f" ("Format String"), w492, w491, w490) -> (resulting string=w493:string)  [unwired: 2 in, 1 out]
        n193 = case shown="\"Read traverse position\"" w477 {
          tunnel: w476 -> [w497 w499]
          tunnel: [w497 w498] -> w475
          frame "Move traverse", Default {
          }
          frame "Read traverse position" {
            n194 = Increment(x=w499) -> (x+1=w498:i32)
          }
        }
        n195 = Select(t="\nThe traverse was probably powered down since the last move. Its position has now been retaught and now all should be well.", s=w485, f="") -> (s? t:f=w486:string)
        n196 = call "Write_out_serial_log.vi"("Header message"=w493) -> ()
        n197 = Concatenate Strings(w481, w486) -> (w478:string)
        n198 = Empty String/Path?(string/path=w478) -> (empty?=w480:bool)
        n199 = Not(x=w480) -> (.not. x?=w479:bool)
      }
      frame 18 {
        # "Add demanded position"
        n200 = case shown="\"Work in Model Coordinates\"" w501 {
          tunnel: w504 -> [_ w519]
          tunnel: w503 -> [w514 w518]
          tunnel: [w514 w516] -> w502
          tunnel: [" (Tunnel Coordinates)" " (Model Coordinates)"] -> w500
          frame "Work in Tunnel Coordinates" {
          }
          frame "Work in Model Coordinates" {
            n201 = call "Coordinate_rotation.vi"("Input Position"=w518, "Coordinate rotation (deg)"=w519, "Mode"=T4."To User Coordinates") -> ("Output Position"=w516:dbl[])
          }
        }
        n202 = for {
          tunnel: w509 -> [w527] mode=indexing
          shift-right: [w522] -> w506
          shift-left: "\nDem Pos " -> [w525]
          tunnel: w502 -> [w520] mode=indexing
          n203 = Unbundle By Name(w527) -> ("Channel Properties.Channel Name"=w526:string)
          n204 = call "Split_Ch_name.vi"("Ch name"=w526) -> ("Low level"=w524:string)  [unwired: 2 out]
          n205 = Format Into String(format string="%s=%.1f, " ("Format String"), w524, w520) -> (resulting string=w521:string)  [unwired: 2 in, 1 out]
          n206 = Concatenate Strings(w525, w521) -> (w522:string)
        }
        n207 = Concatenate Strings(w507, w506, w500) -> (w505:string)
      }
      frame 19 {
        # "Add Achieved Position"
        n208 = local read "Position Output XYZ"() -> (w528:dbl[])
        n209 = case shown="\"Work in Tunnel Coordinates\"" w529 {
          tunnel: w531 -> [_ w545]
          tunnel: [w542 w544] -> w530
          tunnel: w528 -> [w542 w543]
          frame "Work in Tunnel Coordinates" {
          }
          frame "Work in Model Coordinates" {
            n210 = call "Coordinate_rotation.vi"("Input Position"=w543, "Coordinate rotation (deg)"=w545, "Mode"=T4."To User Coordinates") -> ("Output Position"=w544:dbl[])
          }
        }
        n211 = for {
          tunnel: w538 -> [w558] mode=indexing
          shift-right: [w553] -> w535
          shift-left: "\nAchieved Pos " -> [w556]
          tunnel: w530 -> [w551] mode=indexing
          n212 = Unbundle By Name(w558) -> ("Channel Properties.Channel Name"=w557:string)
          n213 = call "Split_Ch_name.vi"("Ch name"=w557) -> ("Low level"=w555:string)  [unwired: 2 out]
          n214 = Format Into String(format string="%s=%.1f, " ("Format String"), w555, w551) -> (resulting string=w552:string)  [unwired: 2 in, 1 out]
          n215 = Concatenate Strings(w556, w552) -> (w553:string)
        }
        n216 = case shown="\"Manual Control\"" w533 {
          tunnel: ["When requesting a move." "When reading position." "When teaching position." "When using manual control."] -> w532
          frame "Move traverse" {
          }
          frame "Read traverse position" {
          }
          frame "Teach Position" {
          }
          frame "Move traverse" {
          }
        }
        n217 = Concatenate Strings(w536, w535, w532) -> (w534:string)
      }
    }
  }
  "Error String" <- w7
